vi "Calculate scan rate.vi"(8 "Scan rate number":dbl, 9 "Number of steps":dbl, 10 "Scan rate max (V/s)":dbl, 11 "Scan rate min (V/s)":dbl) -> (3 "Scan rate":dbl)   [LabVIEW 2011]
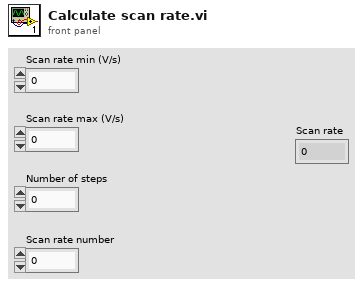
[diagram p1: front panel]
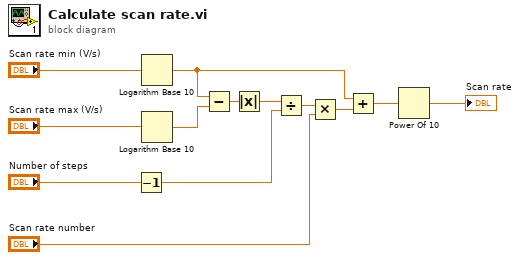
[diagram p0: block diagram]
diagram:
  n1 = Decrement(x="Number of steps") -> (x-1=w7:dbl)
  n2 = Logarithm Base 10(1:"Scan rate min (V/s)") -> (0:w3:dbl)
  n3 = Logarithm Base 10(1:"Scan rate max (V/s)") -> (0:w11:dbl)
  n4 = Subtract(x=w3, y=w11) -> (x-y=w10:dbl)
  n5 = Absolute Value(x=w10) -> (abs(x)=w8:dbl)
  n6 = Divide(x=w8, y=w7) -> (x/y=w6:dbl)
  n7 = Multiply(x=w6, y="Scan rate number") -> (x*y=w4:dbl)
  n8 = Add(x=w3, y=w4) -> (x+y=w2:dbl)
  n9 = Power Of 10(x=w2) -> (10^x=→"Scan rate":dbl)
